vi "Operator Console Controls.vi"   [LabVIEW 2017]
uses:
  <vilib>/Rock Robotics/WPI/Utilities/WPI_GetSetVariantRefNum.vi
  Robot Global Data.vi
types:
  T1 = typedef "WPI_JoystickDevRef.ctl" = cluster{"Device":T2}
  T2 = typedef "WPI_JoystickDeviceEnum.ctl" = enum16{"USB 0", "USB 1", "USB 2", "USB 3", "USB 4", "USB 5"}
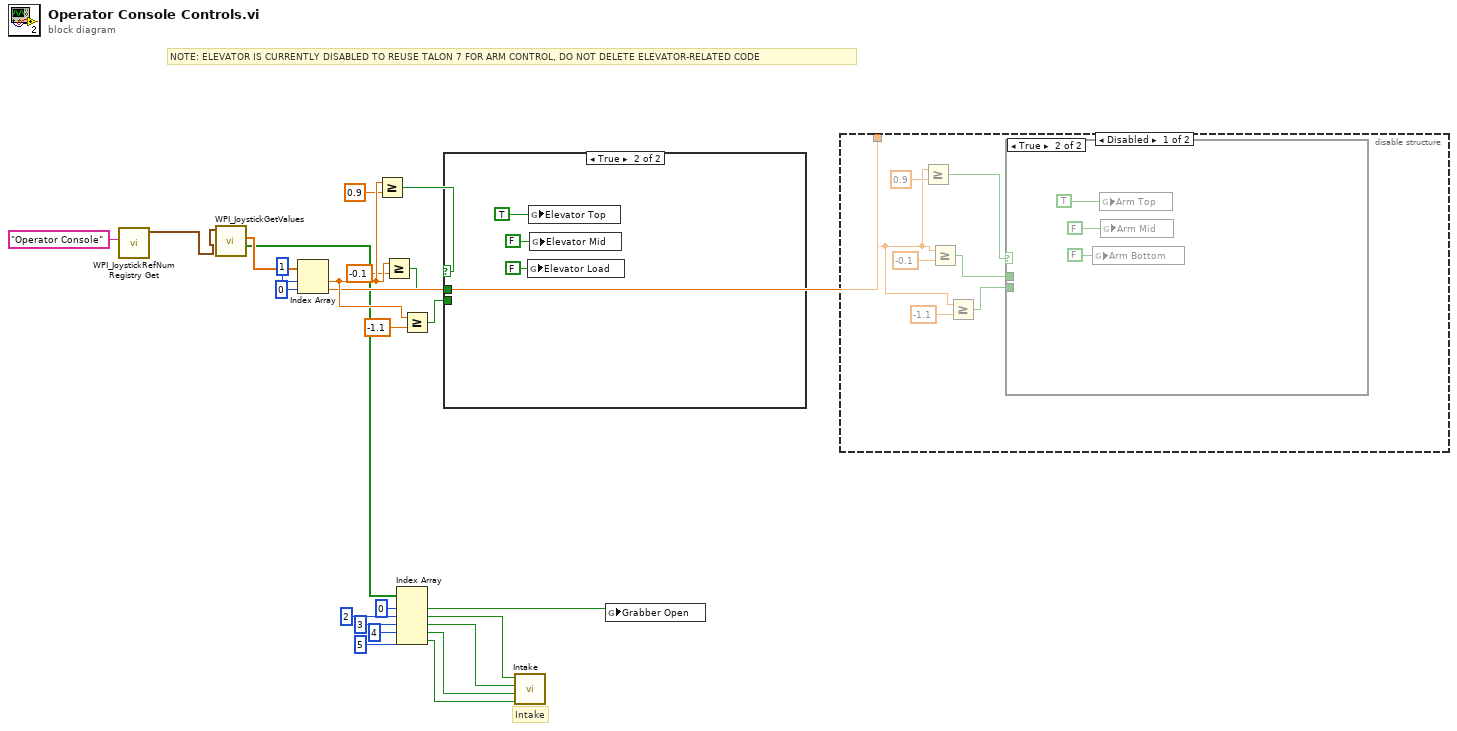
[diagram p0: block diagram]
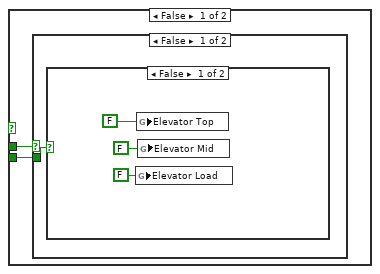
[diagram p2: hidden frame]
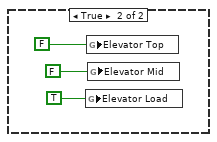
[diagram p3: hidden frame]
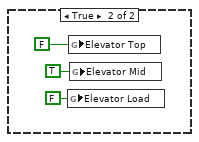
[diagram p4: hidden frame]
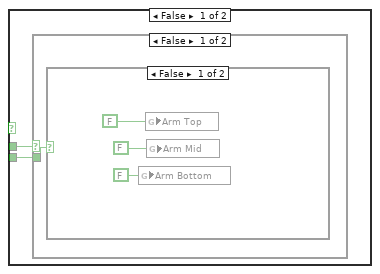
[diagram p5: hidden frame]
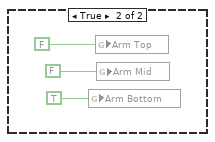
[diagram p6: hidden frame]
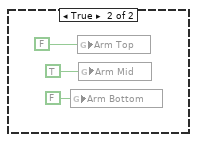
[diagram p7: hidden frame]
diagram:
  # "Intake"
  # "NOTE: ELEVATOR IS CURRENTLY DISABLED TO REUSE TALON 7 FOR ARM CONTROL, DO NOT DELETE ELEVATOR-RELATED CODE"
  n1 = call <vilib>:"WPI_JoystickRefNum Registry Get.vi"("refnum name"="Operator Console") -> ("JoystickDevRef"=w24:T1)  [unwired: 9 in, 1 out]
  n2 = call <vilib>:"WPI_JoystickGetValues.vi"("JoystickDevRef"=w24) -> ("Buttons"=w3:bool[], "Axes"=w22:dbl[])  [unwired: 6 in, 3 out]
  n3 = Index Array(array=w22, index #1=1 ("index"), index #2=0 ("index")) -> (element #1=w21:dbl, element #2=w18:dbl)
  n4 = Greater Or Equal?(x=w21, y=0.9) -> (x >= y?=w16:bool)
  n5 = Greater Or Equal?(x=w21, y=-0.1) -> (x >= y?=w14:bool)
  n6 = Index Array "Index Array"(array=w3, index #1=0 ("index"), index #2=2 ("index"), index #3=3 ("index"), index #4=4 ("index"), index #5=5 ("index")) -> (element #1=w2:bool, element #2=w7:bool, element #3=w6:bool, element #4=w5:bool, element #5=w4:bool)
  n7 = Greater Or Equal?(x=w21, y=-1.1) -> (x >= y?=w12:bool)
  n8 = case shown="True" w16 {
    tunnel: w14 -> [w26 _]
    tunnel: w12 -> [w25 _]
    frame False {
      n9 = case shown="False" w26 {
        tunnel: w25 -> [w27 _]
        frame False {
          n10 = case shown="False" w27 {
            frame False {
              n11 = global write "Robot Global Data.vi" "Elevator Load"(FALSE ("Elevator Mid")) -> ()
              n12 = global write "Robot Global Data.vi" "Elevator Top"(FALSE ("Elevator Bottom")) -> ()
              n13 = global write "Robot Global Data.vi" "Elevator Mid"(FALSE ("Elevator Mid")) -> ()
            }
            frame True {
              n14 = global write "Robot Global Data.vi" "Elevator Load"(TRUE ("Elevator Mid")) -> ()
              n15 = global write "Robot Global Data.vi" "Elevator Top"(FALSE ("Elevator Bottom")) -> ()
              n16 = global write "Robot Global Data.vi" "Elevator Mid"(FALSE ("Elevator Mid")) -> ()
            }
          }
        }
        frame True {
          n17 = global write "Robot Global Data.vi" "Elevator Load"(FALSE ("Elevator Mid")) -> ()
          n18 = global write "Robot Global Data.vi" "Elevator Top"(FALSE ("Elevator Bottom")) -> ()
          n19 = global write "Robot Global Data.vi" "Elevator Mid"(TRUE ("Elevator Mid")) -> ()
        }
      }
    }
    frame True {
      n20 = global write "Robot Global Data.vi" "Elevator Load"(FALSE ("Elevator Mid")) -> ()
      n21 = global write "Robot Global Data.vi" "Elevator Top"(TRUE ("Elevator Bottom")) -> ()
      n22 = global write "Robot Global Data.vi" "Elevator Mid"(FALSE ("Elevator Mid")) -> ()
    }
  }
  n23 = call "Intake.vi"("Intake Out Full"=w4, "Intake Out 1/4"=w5, "Intake In Full"=w6, "Intake In 1/4"=w7) -> ()  [unwired: 8 in]
  n24 = global write "Robot Global Data.vi" "Grabber Open"(w2) -> ()
  n25 = disable-structure shown="Disabled" {
    disable-tunnel: w18 -> [w40 _]
    frame Disabled {
      n26 = Greater Or Equal?(x=w40, y=0.9) -> (x >= y?=w45:bool)
      n27 = Greater Or Equal?(x=w40, y=-0.1) -> (x >= y?=w43:bool)
      n28 = Greater Or Equal?(x=w40, y=-1.1) -> (x >= y?=w41:bool)
      n29 = case shown="True" w45 {
        tunnel: w43 -> [w48 _]
        tunnel: w41 -> [w47 _]
        frame False {
          n30 = case shown="False" w48 {
            tunnel: w47 -> [w49 _]
            frame False {
              n31 = case shown="False" w49 {
                frame False {
                  n32 = global write "Robot Global Data.vi" "Arm Bottom"(FALSE ("Elevator Mid")) -> ()
                  n33 = global write "Robot Global Data.vi" "Arm Top"(FALSE ("Elevator Bottom")) -> ()
                  n34 = global write "Robot Global Data.vi" "Arm Mid"(FALSE ("Elevator Mid")) -> ()
                }
                frame True {
                  n35 = global write "Robot Global Data.vi" "Arm Bottom"(TRUE ("Elevator Mid")) -> ()
                  n36 = global write "Robot Global Data.vi" "Arm Top"(FALSE ("Elevator Bottom")) -> ()
                  n37 = global write "Robot Global Data.vi" "Arm Mid"(FALSE ("Elevator Mid")) -> ()
                }
              }
            }
            frame True {
              n38 = global write "Robot Global Data.vi" "Arm Bottom"(FALSE ("Elevator Mid")) -> ()
              n39 = global write "Robot Global Data.vi" "Arm Top"(FALSE ("Elevator Bottom")) -> ()
              n40 = global write "Robot Global Data.vi" "Arm Mid"(TRUE ("Elevator Mid")) -> ()
            }
          }
        }
        frame True {
          n41 = global write "Robot Global Data.vi" "Arm Bottom"(FALSE ("Elevator Mid")) -> ()
          n42 = global write "Robot Global Data.vi" "Arm Top"(TRUE ("Elevator Bottom")) -> ()
          n43 = global write "Robot Global Data.vi" "Arm Mid"(FALSE ("Elevator Mid")) -> ()
        }
      }
    }
    frame Enabled {
    }
  }
